vi "Initialize LINX Resources.vi"() -> (3 "LINX Resources":T1)   [LabVIEW 2020]
uses:
  Type Definitions/LINX Resources.ctl
  <vilib>/MediaMongrels/LINX Raspberry Pi Addons/LINX SPI/LINX SPI.lvclass
  <vilib>/MediaMongrels/LINX Raspberry Pi Addons/ADS1256 ADC/LINX-ADS1256.lvclass
  <vilib>/MediaMongrels/LINX Raspberry Pi Addons/LINX-DAC8552/LINX-DAC8552.lvclass
  <vilib>/MakerHub/LINX/Private/Type Defs/LINX Ref.ctl
  <vilib>/MakerHub/LINX/Private/Type Defs/Platform.ctl
  <vilib>/MakerHub/LINX/Private/Type Defs/Interface.ctl
  <vilib>/MakerHub/LINX/Private/Device/Type Defs/LINX Device Config.ctl
  <vilib>/MakerHub/LINX/Private/Device/Type Defs/TCP Config.ctl
  <vilib>/MakerHub/LINX/Private/Device/Type Defs/Channels.ctl
  <vilib>/MakerHub/LINX/Public/Peripherals/SPI/SPI CS Config.ctl
  <vilib>/MakerHub/LINX/Private/Type Defs/Peripherals/SPI/SPI CS Logic Level.ctl
  <vilib>/MakerHub/LINX/Private/Type Defs/Peripherals/SPI/SPI Configuration.ctl
  <vilib>/MakerHub/LINX/Private/Type Defs/Peripherals/SPI/SPI Bit Order.ctl
  <vilib>/MakerHub/LINX/Private/Type Defs/Peripherals/SPI/SPI Mode.ctl
  <vilib>/MediaMongrels/LINX Raspberry Pi Addons/ADS1256 ADC/Programmable Gain Selection.ctl
  <vilib>/MediaMongrels/LINX Raspberry Pi Addons/ADS1256 ADC/Sample Rate.ctl
  <vilib>/MakerHub/LINX/Public/Utilities/Open Local.vi
  <vilib>/MakerHub/LINX/LMH-LINX.lvlib
  <vilib>/MakerHub/LINX/Private/Device/Device.lvlib
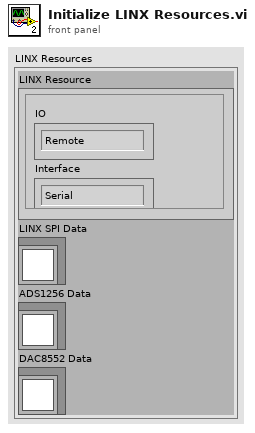
[diagram p1: front panel]
types:
  T1 = typedef "LINX Resources.ctl" = cluster{"LINX Resource":T2, "LINX SPI Data":refnum<class "LINX SPI.lvclass">, "ADS1256 Data":refnum<class "LINX-ADS1256.lvclass">, "DAC8552 Data":refnum<class "LINX-DAC8552.lvclass">}
  T2 = typedef "LMH-LINX.lvlib/LINX Ref.ctl" = cluster{"IO":T3, "Interface":T4, "LINX Device Config":T5}
  T3 = typedef "LMH-LINX.lvlib/Platform.ctl" = enum16{"Remote", "Local"}
  T4 = typedef "LMH-LINX.lvlib/Interface.ctl" = enum16{"Serial", "TCP"}
  T5 = typedef "LMH-LINX.lvlib/Device.lvlib/LINX Device Config.ctl" = cluster{"Interface":T4, "COM Port":refnum<visa-resource-name>, "TCP Configuration":T6, "Device Family":u8, "Device ID":u8, "Device Name":string, "TCP Ref":refnum<k5>, "Channels":T7}
  T6 = typedef "LMH-LINX.lvlib/Device.lvlib/TCP Config.ctl" = cluster{"IP Address":string, "Port":u16}
  T7 = typedef "LMH-LINX.lvlib/Channels.ctl" = cluster{"DI":u8[], "DO":u8[], "AI":u8[], "AO":u8[], "PWM":u8[], "QE":u8[], "UART":u8[], "I2C 2":u8[], "SPI":u8[], "CAN":u8[], "Servo":u8[], "AI Ref (V)":dbl, "AI Resolution (Bits)":u8, "AO Ref (V)":dbl, "AO Resolution (Bits)":u8}
  T8 = typedef "LINX-ADS1256.lvclass/Sample Rate.ctl" = enum16{"2.5Hz", "5Hz", "10Hz", "15Hz", "25Hz", "30Hz", "50Hz", "60Hz", "100Hz", "500Hz", "1000Hz", "2000Hz", "3750Hz", "7500Hz", "15000Hz", "30000Hz"}
  T9 = typedef "LINX-ADS1256.lvclass/Programmable Gain Selection.ctl" = enum16{"+/-5V (1)", "+/-2.5V (2)", "+/-1.25V (4)", "+/-0.625V (8)", "+/-312.5mV (16)", "+/-156.25mV (32)", "+/-78.125mV (64)"}
  T10 = typedef "LMH-LINX.lvlib/SPI Configuration.ctl" = cluster{"Clock Frequency":u32, "Bit Order":T11, "SPI Mode":T12}
  T11 = typedef "LMH-LINX.lvlib/SPI Bit Order.ctl" = enum8{"LSb First", "MSb First"}
  T12 = typedef "LMH-LINX.lvlib/SPI Mode.ctl" = enum8{"Mode 0", "Mode 1", "Mode 2", "Mode 3"}
  T13 = typedef "LMH-LINX.lvlib/SPI CS Config.ctl" = cluster{"CS Channel":u8, "CS Logic Level":T14}
  T14 = typedef "LMH-LINX.lvlib/SPI CS Logic Level.ctl" = enum8{"Active Low", "Active High"}
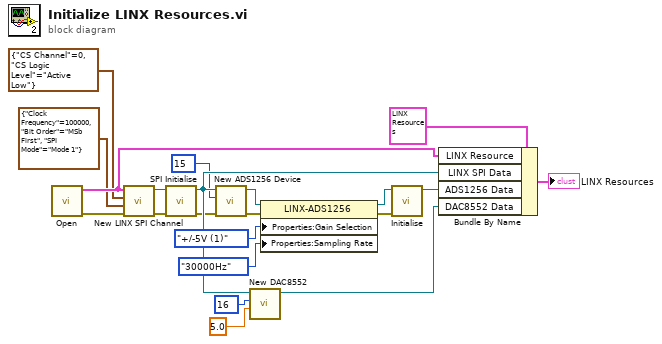
[diagram p0: block diagram]
diagram:
  n1 = call-poly <vilib>:"Open.vi"() -> ("Error Out"=w13:errorcluster, "LINX Resource"=w17:T2)  [unwired: 9 in, 1 out]
  n2 = call <vilib>:"New LINX SPI Channel.vi"("error in (no error)"=w13, "SPI Configuration"=T10 {"Clock Frequency"=100000, "Bit Order"=enum."MSb First", "SPI Mode"=enum."Mode 1"}, "CS Configuration"=T13 {"CS Channel"=0, "CS Logic Level"=enum."Active Low"}, "LINX Resource"=w17) -> ("error out"=w9:errorcluster, "LINX SPI out"=w10:refnum<class "LINX SPI.lvclass">)  [unwired: 6 in]
  n3 = call-dynamic "SPI Initialise.vi"("error in (no error)"=w9, "LINX SPI in"=w10) -> ("error out"=w8:errorcluster, "LINX SPI out"=w18:refnum<class "LINX SPI.lvclass">)  [unwired: 8 in]
  n4 = call <vilib>:"New ADS1256 Device.vi"("error in (no error)"=w8, "SPI CS Line"=u8 15 ("I2C Slave Address (0x48)"), "SPI"=w18) -> ("error out"=w6:errorcluster, "LINX-ADS1X15 out"=w4:refnum<class "LINX-ADS1256.lvclass">)  [unwired: 7 in]
  n5 = call <vilib>:"New DAC8552.vi"("VRef (5V)"=5.0, "SPI CS Line"=u8 16, "SPI in"=w18) -> ("LINX-DAC8552 out"=w20:refnum<class "LINX-DAC8552.lvclass">)  [unwired: 7 in, 1 out]
  n6 = property class="LINX-ADS1256"(reference=w4, error in=w6, "Properties:Gain Selection"=Programmable_Gain_Selection."+/-5V (1)" ("Gain Selection"), "Properties:Sampling Rate"=Sample_Rate."30000Hz" ("Sampling Rate")) -> (reference out=w3:refnum<class "LINX-ADS1256.lvclass">, error out=w5:errorcluster)
  n7 = call <vilib>:"Initialise.vi"("error in (no error)"=w5, "LINX-ADS1256 in"=w3) -> ("LINX-ADS1256 out"=w19:refnum<class "LINX-ADS1256.lvclass">)  [unwired: 8 in, 1 out]
  n8 = Bundle By Name(cluster=T1 {"LINX Resource"={"IO"=enum."Remote", "Interface"=enum."Serial", "LINX Device Config"={"Interface"=enum."Serial", "COM Port"="", "TCP Configuration"={"IP Address"="", "Port"=0}, "Device Family"=0, "Device ID"=0, "Device Name"="", "TCP Ref"=refnum, "Channels"={"DI"=[], "DO"=[], "AI"=[], "AO"=[], "PWM"=[], "QE"=[], "UART"=[], "I2C 2"=[], "SPI"=[], "CAN"=[], "Servo"=[], "AI Ref (V)"=0.0, "AI Resolution (Bits)"=0, "AO Ref (V)"=0.0, "AO Resolution (Bits)"=0}}}, "LINX SPI Data"=refnum, "ADS1256 Data"=refnum, "DAC8552 Data"=refnum}, "LINX Resource"=w17, "LINX SPI Data"=w18, "ADS1256 Data"=w19, "DAC8552 Data"=w20) -> (→"LINX Resources":T1)
